vi "CalculateInputString.vi"(1 "InputStrings":string) -> (0 "Result":dbl)   [LabVIEW 2016]
uses:
  <vilib>/regexp/Match Regular Expression.xnode
panel:
  out "TempAns":dbl
  in  "ArrayOfAvailableOperators":cluster{"Chars":string, "Boolean":bool}[](array[cluster])=[{"Chars"="+", "Boolean"=FALSE}, {"Chars"="-", "Boolean"=FALSE}, {"Chars"="*", "Boolean"=FALSE}, {"Chars"="/", "Boolean"=FALSE}, {"Chars"="^", "Boolean"=FALSE}]
  out "ArrayOfOperators":string[](array[string])
  out "ArrayOfDigits":string[](array[string])
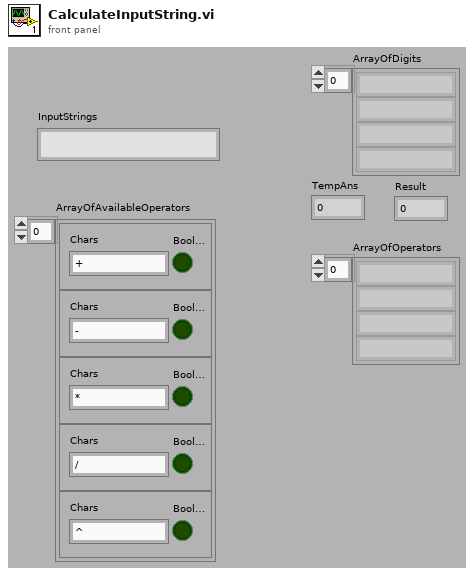
[diagram p1: front panel]
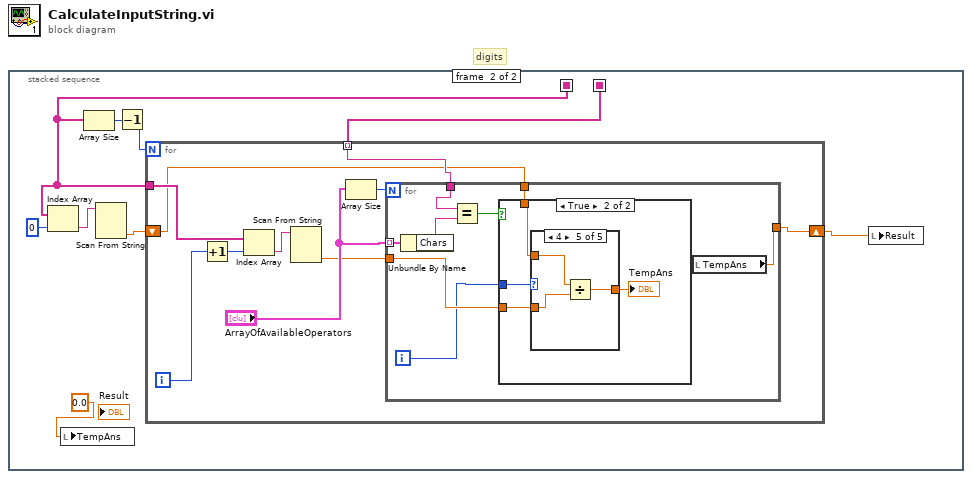
[diagram p0: block diagram]
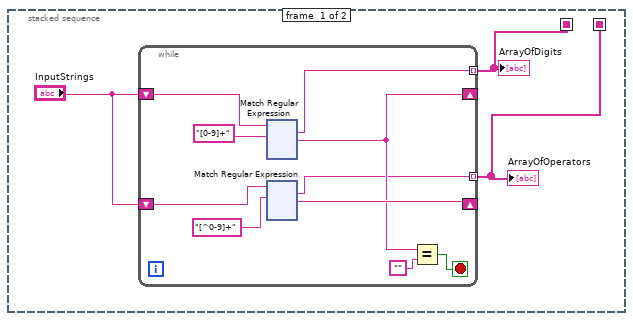
[diagram p2: hidden frame]
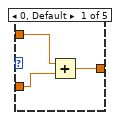
[diagram p4: hidden frame]
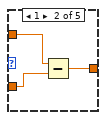
[diagram p5: hidden frame]
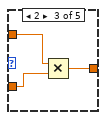
[diagram p6: hidden frame]
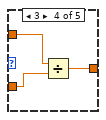
[diagram p7: hidden frame]
diagram:
  # "digits"
  n1 = stacked-sequence {
    seq-local: [w2 _] -> [_ w240]
    seq-local: [w1 _] -> [_ w242]
    frame #0 {
      n2 = while {
        shift-right: [w6] -> _
        shift-left: "InputStrings" -> [w12]
        tunnel: [w11] -> w2 mode=indexing
        shift-right: [w8] -> _
        shift-left: "InputStrings" -> [w9]
        tunnel: [w4] -> w1 mode=indexing
        stop <- w7 stop-if-true
        n3 = xnode "Match Regular Expression"("input string"=w12, "regular expression"="[0-9]+") -> ("whole match"=w11:string, "after match"=w6:string)  [unwired: 4 in, 3 out]
        n4 = xnode "Match Regular Expression"("input string"=w9, "regular expression"="[^0-9]+") -> ("whole match"=w4:string, "after match"=w8:string)  [unwired: 4 in, 3 out]
        n5 = Equal?(x=w6, y="") -> (x = y?=w7:bool)
      }
      "ArrayOfDigits" <- w2
      "ArrayOfOperators" <- w1
    }
    frame #1 {
      n6 = Index Array(array=w240, index=0) -> (element=w241:string)
      n7 = local write "TempAns"(0.0) -> ()
      n8 = Array Size(array=w240) -> (size(s)=w244:i32)
      n9 = Scan From String(input string=w241) -> (output 1=w238:dbl)  [unwired: 4 in, 3 out]
      n10 = Decrement(x=w244) -> (x-1=w243:i32)
      n11 = for {
        N: w243 -> [_]
        tunnel: w240 -> [w254]
        tunnel: w242 -> [w249] mode=indexing
        shift-right: [w245] -> w236
        shift-left: w238 -> [w246]
        i -> [w252]
        n12 = Increment(x=w252) -> (x+1=w253:i32)
        n13 = Index Array(array=w254, index=w253) -> (element=w248:string)
        n14 = Scan From String(input string=w248) -> (output 1=w247:dbl)  [unwired: 4 in, 3 out]
        n15 = Array Size(array="ArrayOfAvailableOperators") -> (size(s)=w251:i32)
        n16 = for {
          N: w251 -> [_]
          tunnel: "ArrayOfAvailableOperators" -> [w261] mode=indexing
          tunnel: w249 -> [w262]
          tunnel: w246 -> [w258]
          tunnel: w247 -> [w257]
          tunnel: [w255] -> w245
          i -> [w256]
          n17 = Unbundle By Name(w261) -> ("Chars"=w260:string)
          n18 = Equal?(x=w262, y=w260) -> (x = y?=w259:bool)
          n19 = case shown="True" w259 {
            tunnel: w256 -> [_ w266]
            tunnel: w258 -> [_ w265]
            tunnel: w257 -> [_ w264]
            frame False {
            }
            frame True {
              n20 = case shown="4" w266 {
                tunnel: w265 -> [w269 w272 w275 w278 w281]
                tunnel: w264 -> [w268 w271 w274 w277 w280]
                tunnel: [w267 w270 w273 w276 w279] -> w263
                frame 0, Default {
                  n21 = Add(x=w269, y=w268) -> (x+y=w267:dbl)
                }
                frame 1 {
                  n22 = Subtract(x=w272, y=w271) -> (x-y=w270:dbl)
                }
                frame 2 {
                  n23 = Multiply(x=w275, y=w274) -> (x*y=w273:dbl)
                }
                frame 3 {
                  n24 = Divide(x=w278, y=w277) -> (x/y=w276:dbl)
                }
                frame 4 {
                  n25 = Divide(x=w281, y=w280) -> (x/y=w279:dbl)
                }
              }
              "TempAns" <- w263
            }
          }
          n26 = local read "TempAns"() -> (w255:dbl)
        }
      }
      n27 = local write "Result"(w236) -> ()
    }
  }
